vi "MasterAcquisitionFile_PCO_IOS_SingleWavelength.vi"() -> ()   [LabVIEW 2020]
uses:
  <userlib>/PCO LabVIEW 5.0.0/pco.camera/Controls/binning.ctl
  <vilib>/vision/driver/IMAQdx.llb/IMAQdx Camera Control Mode.ctl
  <vilib>/vision/driver/IMAQdx.llb/IMAQdx Acquisition Mode.ctl
  <vilib>/userDefined/High Color/IMAQdx.ctl
  <userlib>/PCO LabVIEW 5.0.0/pco.camera/Camera.lvclass
  <vilib>/vision/driver/IMAQdx.llb/IMAQdx Buffer Number Mode.ctl
  <vilib>/DAQmx/write.llb/DAQmx Write (Digital 1D Wfm NChan NSamp).vi
  <vilib>/DAQmx/read.llb/DAQmx Read (Analog 1D Wfm NChan NSamp).vi
  <vilib>/Waveform/DWDTOps.llb/DWDT Digital to Boolean Array.vi
  <vilib>/DAQmx/create/channels.llb/DAQmx Create Channel (CO-Pulse Generation-Frequency).vi
  <vilib>/DAQmx/configure/timing.llb/DAQmx Timing (Implicit).vi
  <vilib>/DAQmx/create/channels.llb/DAQmx Create Channel (AI-Voltage-Basic).vi
  <vilib>/DAQmx/configure/timing.llb/DAQmx Timing (Sample Clock).vi
  <vilib>/DAQmx/configure/trigger.llb/DAQmx Start Trigger (Digital Edge).vi
  <vilib>/DAQmx/create/channels.llb/DAQmx Create Channel (DO-Digital Output).vi
  <vilib>/Waveform/DWDTOps.llb/DWDT Boolean Array to Digital.vi
  <vilib>/Waveform/DWDTOps.llb/DWDT Uncompress Digital.vi
  <vilib>/DAQmx/miscellaneous.llb/DAQmx Fill In Error Info.vi
  <vilib>/vision/driver/NI_Vision_Acquisition_Software.lvlib
  <resource>/objmgr/imaqdx.rc
  <resource>/objmgr/daqmx.rc
panel:
  out "Recorded Images":u32
  in  "ROI":cluster{"x0":u64, "y0":u64, "x1":u64, "y1":u64}={"x0"=1, "y0"=1, "x1"=640, "y1"=540}
  in  "Binning":T1={"vert"=4, "horz"=4}
  in  "TriggerMode":T2(ring)=enum."external exposure start"
  in  "Exposure [s]":dbl=0.01 min=0.0005 max=2.0 step=0.001
  out "Image":T3(plugin-control)
  out "LED":bool
  out "Auditory":bool
  out "RPad":bool
  out "LPad":bool
  out "Finished":bool
  in  "Generate Stimuli":bool=TRUE
  in  "Sol Stim Parameters":cluster{"Fs":dbl, "Samples":dbl}
  in  "LED Stim Parameters":cluster{"Fs":dbl, "Samples":dbl}
  in  "Sol Duty Cycle (%)":dbl=50.0
  in  "Sol Freq":dbl=1.0
  in  "Sol Dur (s)":dbl=1.0
  in  "LED Duty Cycle (%)":dbl=10.0
  in  "LED Freq":dbl=10.0
  in  "LED Dur (s)":dbl=2.0
  out "Stimulus Order":digitalwaveform[](graph)=[{"t0"=timestamp(0 s since 1904-01-01), "dt"=5e-05, "Y"={"transitions"=[], "data"=array6001000x1[6001000 elements]}}, {"t0"=timestamp(0 s since 1904-01-01), "dt"=5e-05, "Y"={"transitions"=[], "data"=array6001000x1[6001000 elements]}}, {"t0"=timestamp(0 s since 1904-01-01), "dt"=5e-05, "Y"={"transitions"=[], "data"=array6001000x1[6001000 elements]}}, {"t0"=timestamp(0 s since 1904-01-01), "dt"=5e-05, "Y"={"transitions"=[], "data"=array6001000x1[6001000 elements]}}]
  out "Solenoid Stim":digitalwaveform(graph)={"t0"=timestamp(0 s since 1904-01-01), "dt"=5e-05, "Y"={"transitions"=[], "data"=array20000x1[20000 elements]}}
  in  "Trial Offset (s)":dbl=5.0
  in  "Interstim (s)":dbl=10.0
  in  "Right Pad":dbl=1.0
  in  "Left Pad":dbl=1.0
  in  "Auditory":dbl=1.0
  in  "LED":dbl
  out "?":T3(plugin-control)
  out "?":T3(plugin-control)
  out "?":T3(plugin-control)
  in  "stop":bool
  out "PCO":bool
  out "Pupil Cam":bool
  out "Whisk Cam":bool
  out "Web Cam":bool
  out "Analog":bool
  out "Web Cam Fs":dbl(knob) scale=0.0..200.0
  out "Whisk Cam Fs":dbl(knob) scale=0.0..200.0
  out "Last Whisk\nBuffer 2":u32=1
  out "Pupil Cam Fs":dbl(knob) scale=0.0..200.0
  out "Dropped 2":u32(slide) caption="Pupil Cam" scale=0.0..99.0
  out "Dev1 Samples":i32
  in  "Dev1 Analog Channels":string[](array[string])=["Cortical_LH", "Force_Sensor", "LPadSol", "RPadSol", "AudSol", "Hippocampus", "EMG", "Cortical_RH", "OptoLED"]
  in  "Analog Acquisition":cluster{"Analog Fs":u16}={"Analog Fs"=20000} {"Analog Fs" format="%0.0f"}
  in  "Sampling Rates":T4={"CBV Cam Fs"=30, "Whisk Cam Fs"=150, "Web Cam Fs"=30, "Pupil Cam Fs"=30}
  out "Notes Size":i32=8
  out "Notes Reversed":string[](array[string])=["Experimenter", "Animal ID", "Hemisphere", "Solenoid PSI", "Isoflurane time", "Session ID", "Amplifier Gain", "LED power (mW)"]
  out "Notes Array":string[](array[string])=["LED power (mW)", "Amplifier Gain", "Session ID", "Isoflurane time", "Solenoid PSI", "Hemisphere", "Animal ID", "Experimenter"]
  in  "Notes:":T5={"Experimenter"="Kevin", "Animal ID"="FS28", "Hemisphere"="LH", "Solenoid PSI"="10", "Isoflurane time"="1420", "Session ID"="Imaging Session One", "Amplifier Gain"="10000", "Opto LED (mW)"="10", "Wavelengths"="530 nm", "Lens mag"="1.5X"}
  in  "Target Path":path=path "D:/FS28/5 minute 530 only" caption="Final Save Location"
  out "Dropped":u32(slide) caption="Whisk Cam" scale=0.0..999.0
  out "Filename":string="230405_14_53_47"
  out "CBV Camera":bool=TRUE
  out "Time Elapsed (Min)":cluster{dbl, dbl}(slide)={15.0, 5.0010000000000004e-05} scale=0.0..15.0 scale format="%.1g"
  in  "Time (min)":dbl(knob)=15.0 min=0.5 max=20.0 step=0.5 scale=0.0..20.0 scale format="%#_2g"
  in  "Temp Path":path=path "D:/LabVIEW Streamed Data" caption="Temporary Path for Streamed Data"
  out "Last Whisk\nBuffer":u32=1
  # "PCO Parameters"
  # "Stimuli"
  # "LPAD"
  # "RPAD"
  # "AUD"
  # "LED"
  # "Dropped Frames"
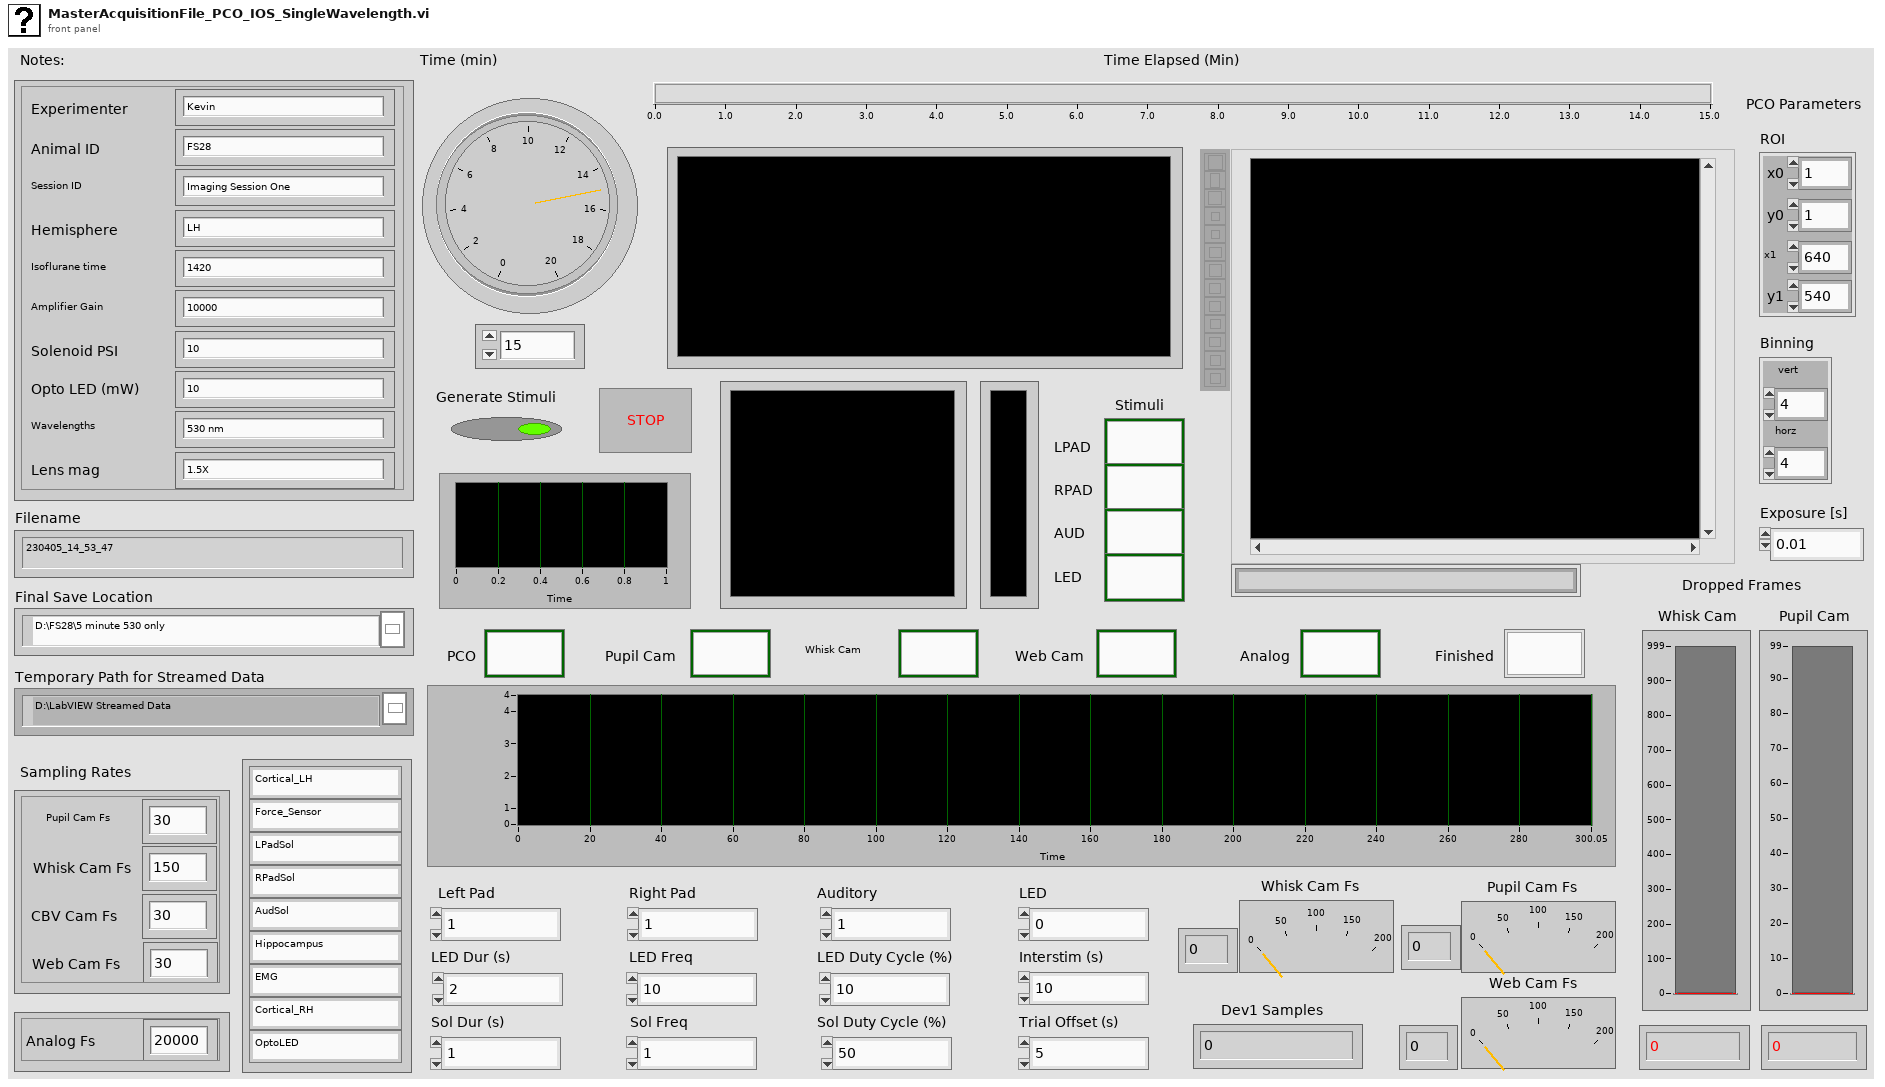
[diagram p1: front panel]
types:
  T1 = typedef "Camera.lvclass/binning.ctl" = cluster{"vert":u16, "horz":u16}
  T2 = enum16{"auto sequence", "software trigger", "external exposure start", "external exposure control"}
  T3 = typedef "IMAQ Image.ctl" = refnum<image>
  T4 = cluster{"CBV Cam Fs":u16, "Whisk Cam Fs":u16, "Web Cam Fs":u16, "Pupil Cam Fs":u16}
  T5 = cluster{"Experimenter":string, "Animal ID":string, "Hemisphere":string, "Solenoid PSI":string, "Isoflurane time":string, "Session ID":string, "Amplifier Gain":string, "Opto LED (mW)":string, "Wavelengths":string, "Lens mag":string}
  T6 = typedef "Image Type" = u32
  T7 = typedef "IMAQdx.ctl" = refnum<k21>
  T8 = enum16{"open", "replace", "create", "open or create", "replace or create", "replace or create with confirmation"}
  T9 = typedef "NI_Vision_Acquisition_Software.lvlib/IMAQdx Acquisition Mode.ctl" = enum32{"One Shot", "Continuous"}
  T10 = typedef "NI_Vision_Acquisition_Software.lvlib/IMAQdx Camera Control Mode.ctl" = enum32{"Controller", "Listener"}
  T11 = enum16{"open", "open or create", "create or replace", "create", "open (read-only)"}
  T12 = cluster{"exposure_time_s":dbl, "delay_time_s":dbl, "roi":cluster{"x0":u64, "y0":u64, "x1":u64, "y1":u64}, "timestamp_mode":u16, "pixelrate":u32, "trigger_mode":u16, "acquire_mode":u16, "metadata_mode":u16, "noisefilter_mode":u16, "binning":T1}
  T13 = typedef "IMAQ AVI2 Refnum.ctl" = refnum<k20>
  T14 = enum16{"sequence", "sequence non blocking", "ring buffer", "fifo", "sequence_dpcore", "sequence_non_blocking_dpcore", "ring_buffer_dpcore", "fifo_dpcore", "tif", "multitif", "pcoraw", "b16", "dicom", "multidicom"}
  T15 = enum16{"Undefined", "Mono8", "Mono16", "BGRA8", "RGBA8", "BGRA16", "RGBA16", "CompressedMono8"}
  T16 = enum16{"big-endian, network order", "native, host order", "little-endian"}
  T17 = typedef "NI_Vision_Acquisition_Software.lvlib/IMAQdx Buffer Number Mode.ctl" = enum32{"Next", "Last", "Buffer Number", "Every", "Last New"}
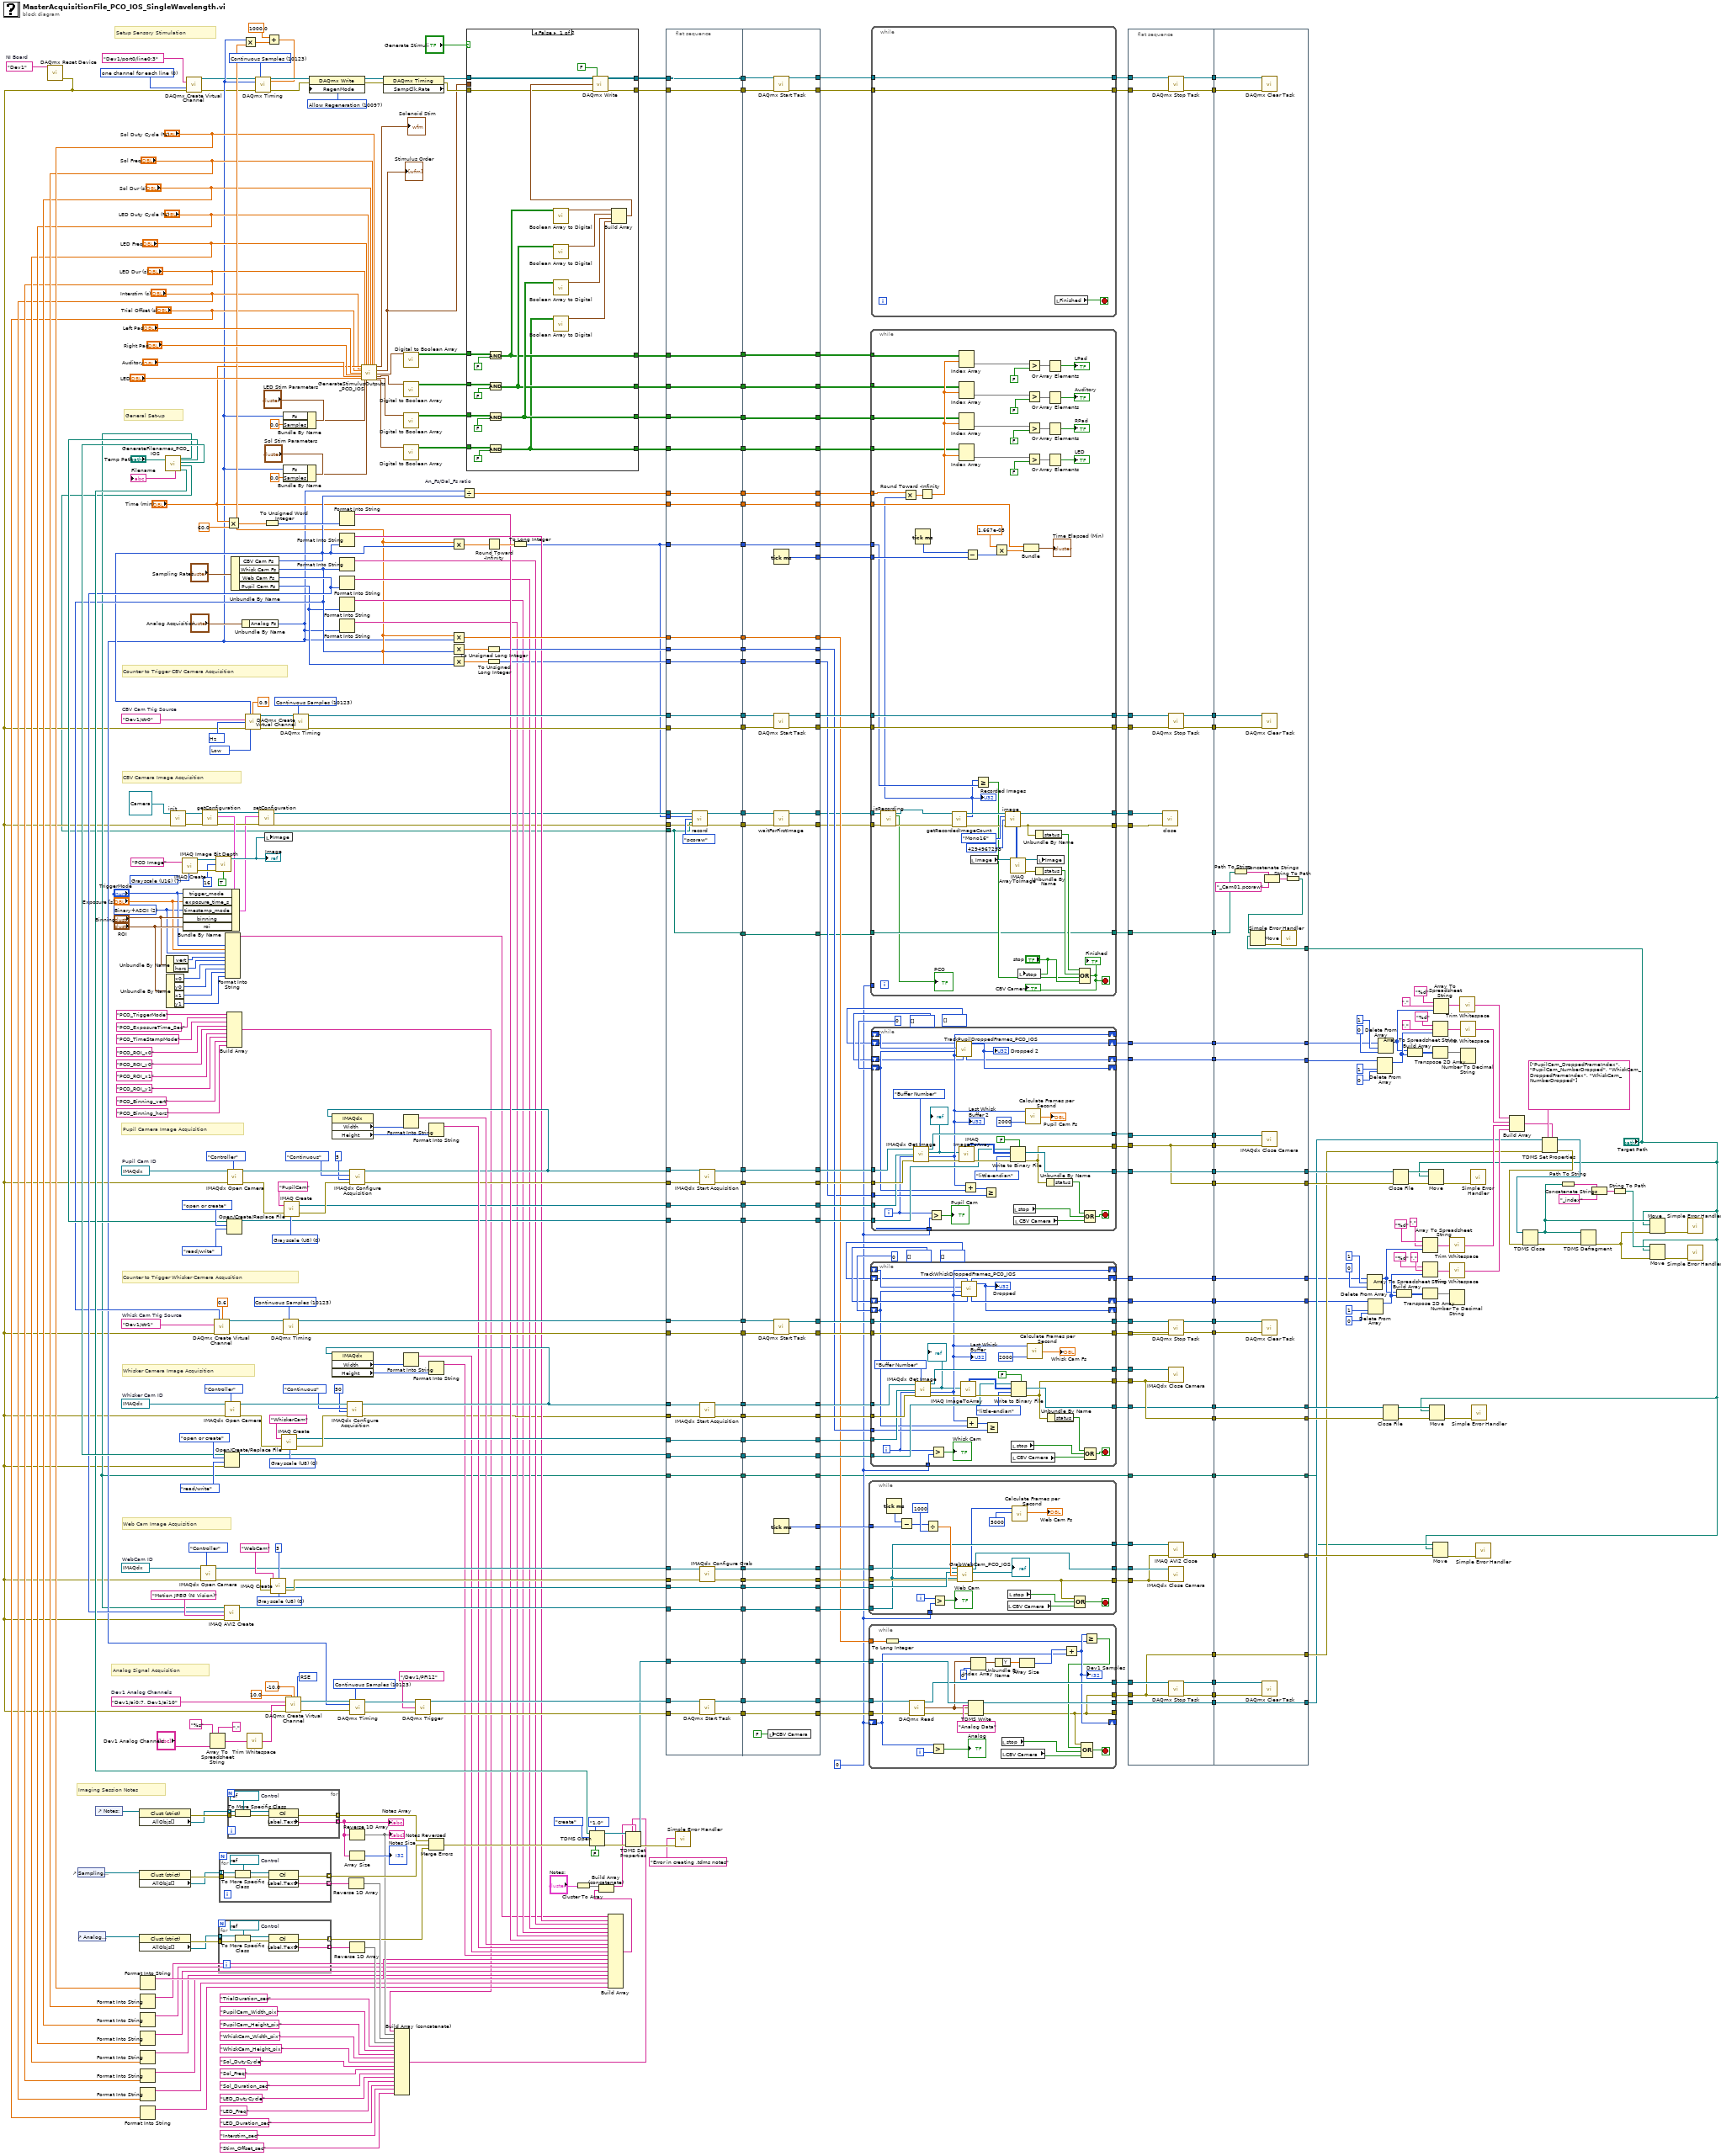
[diagram p0: block diagram]
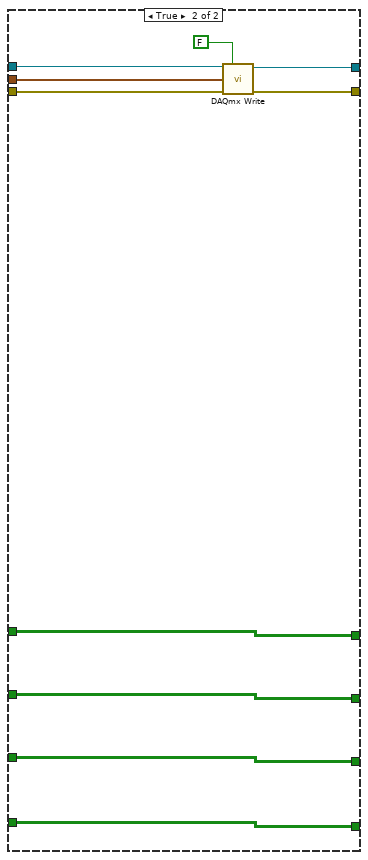
[diagram p2: hidden frame]
diagram:
  w24 = u16 2 items=["OFF", "Binary", "Binary+ASCII", "ASCII"] ("wTimeStampMode")
  w49 = T6 7 items=["Grayscale (U8)", "Grayscale (I16)", "Grayscale (SGL)", "Complex (CSG)", "RGB (U32)", "HSL (U32)", "RGB (U64)", "Grayscale (U16)"] ("Image Type")
  w141 = 10097 items=["Allow Regeneration"=10097, "Do Not Allow Regeneration"=10158] ("RegenMode")
  w142 = 10123 items=["Finite Samples"=10178, "Continuous Samples"=10123, "Hardware Timed Single Point"=12522] ("sample mode")
  w145 = 0 items=["one channel for each line", "one channel for all lines"] ("line grouping")
  w314 = tag "Dev1/ai0:7, Dev1/ai10"  # Dev1 Analog Channels
  w317 = T7 "cam3"  # WebCam ID
  w303 = T7 "cam1"  # Whisker Cam ID
  w441 = tag "Dev1/ctr1"  # Whisk Cam Trig Source
  w265 = T7 "cam2"  # Pupil Cam ID
  w107 = tag "Dev1/ctr0"  # CBV Cam Trig Source
  w268 = T6 0 items=["Grayscale (U8)", "Grayscale (I16)", "Grayscale (SGL)", "Complex (CSG)", "RGB (U32)", "HSL (U32)", "RGB (U64)", "Grayscale (U16)"] ("Image Type")
  w198 = 0
  w386 = 10123 items=["Finite Samples"=10178, "Continuous Samples"=10123, "Hardware Timed Single Point"=12522] ("sample mode")
  w389 = 10083 items=["default"=-1, "RSE"=10083, "NRSE"=10078, "Differential"=10106, "Pseudodifferential"=12529] ("input terminal configuration")
  w424 = T6 0 items=["Grayscale (U8)", "Grayscale (I16)", "Grayscale (SGL)", "Complex (CSG)", "RGB (U32)", "HSL (U32)", "RGB (U64)", "Grayscale (U16)"] ("Image Type")
  w431 = tag "Dev1"  # NI Board
  w432 = 10123 items=["Finite Samples"=10178, "Continuous Samples"=10123, "Hardware Timed Single Point"=12522] ("sample mode")
  w435 = 10373 items=["Hz"=10373] ("units")
  w436 = 10214 items=["High"=10192, "Low"=10214] ("idle state")
  w437 = 10123 items=["Finite Samples"=10178, "Continuous Samples"=10123, "Hardware Timed Single Point"=12522] ("sample mode")
  w444 = T6 0 items=["Grayscale (U8)", "Grayscale (I16)", "Grayscale (SGL)", "Complex (CSG)", "RGB (U32)", "HSL (U32)", "RGB (U64)", "Grayscale (U16)"] ("Image Type")
  # "General Set-up"
  # "Pupil Camera Image Acquisition"
  # "Whisker Camera Image Acquisition"
  # "Imaging Session Notes"
  # "Setup Sensory Stimulation"
  # "CBV Camera Image Acquisition"
  # "Counter to Trigger CBV Camera Acquisition"
  # "Counter to Trigger Whisker Camera Acqusition"
  # "Web Cam Image Acquisition"
  # "Analog Signal Acquisition"
  n1 = call <vilib>:"DAQmx Reset Device.vi"("device in"=w431) -> ("error out"=w39:errorcluster)  [unwired: 14 in]
  n2 = control-ref of="Sampling Rates"() -> (w323:refnum<vi>)
  n3 = control-ref of="Analog Acquisition"() -> (w322:refnum<vi>)
  n4 = control-ref of="Notes:"() -> (w344:refnum<vi>)
  n5 = property class="Clust (strict)"(reference=w344) -> (error out=w347:errorcluster, "AllObjs[]"=w281:refnum<vi>[])  [unwired: 1 in, 1 out]
  n6 = property class="Clust (strict)"(reference=w323) -> (error out=w342:errorcluster, "AllObjs[]"=w282:refnum<vi>[])  [unwired: 1 in, 1 out]
  n7 = property class="Clust (strict)"(reference=w322) -> (error out=w321:errorcluster, "AllObjs[]"=w280:refnum<vi>[])  [unwired: 1 in, 1 out]
  n8 = Format Into String("Sol Duty Cycle (%)") -> (resulting string=w175:string)  [unwired: 3 in, 1 out]
  n9 = Format Into String("Sol Freq") -> (resulting string=w174:string)  [unwired: 3 in, 1 out]
  n10 = Format Into String("Sol Dur (s)") -> (resulting string=w173:string)  [unwired: 3 in, 1 out]
  n11 = Format Into String("LED Duty Cycle (%)") -> (resulting string=w172:string)  [unwired: 3 in, 1 out]
  n12 = Format Into String("LED Freq") -> (resulting string=w171:string)  [unwired: 3 in, 1 out]
  n13 = Format Into String("LED Dur (s)") -> (resulting string=w170:string)  [unwired: 3 in, 1 out]
  n14 = Format Into String("Interstim (s)") -> (resulting string=w169:string)  [unwired: 3 in, 1 out]
  n15 = Format Into String("Trial Offset (s)") -> (resulting string=w168:string)  [unwired: 3 in, 1 out]
  n16 = call "GenerateFilenames_PCO_IOS.vi"("path"="Temp Path") -> ("TDMS Path"=w339:path, "PCO Path"=w5:path, "Basler Path"=w427:path, "WebCam Path"=w53:path, "Analog file name"=→"Filename":string, "Basler2 Path"=w264:path)  [unwired: 3 in, 2 out]
  n17 = Unbundle By Name("Binning") -> ("vert"=w23:u16, "horz"=w22:u16)
  n18 = Unbundle By Name("ROI") -> ("x0"=w21:u64, "y0"=w20:u64, "x1"=w19:u64, "y1"=w18:u64)
  n19 = call-dynamic "init.vi"("Camera in"=refnum<class "Camera.lvclass"> refnum ("PCOCamera in"), "error in (no error)"=w39) -> ("Camera out"=w42:refnum<class "Camera.lvclass">, "error out"=w41:errorcluster)  [unwired: 7 in]
  n20 = call "IMAQ Create"("Image Name"="PCO Image", "Image Type"=w49) -> ("New Image"=w48:T3, "error out"=w47:errorcluster)  [unwired: 3 in]
  n21 = call-poly <vilib>:"DAQmx Create Virtual Channel.vi"("lines"=tag "Dev1/port0/line0:3", "line grouping"=w145, "error in"=w39) -> ("task out"=w144:refnum<k21>, "error out"=w143:errorcluster)  [unwired: 11 in]
  n22 = call <vilib>:"IMAQdx Open Camera.vi"("Camera Control Mode"=IMAQdx_Camera_Control_Mode."Controller", "error in"=w39, "Session In"=w317) -> ("error out"=w420:errorcluster, "Session Out"=w418:T7)  [unwired: 7 in]
  n23 = call-dynamic "getConfiguration.vi"("error in (no error)"=w41, "Camera in"=w42) -> ("error out"=w40:errorcluster, "configuration"=w44:T12, "Camera out"=w43:refnum<class "Camera.lvclass">)  [unwired: 7 in]
  n24 = Bundle By Name(cluster=w44, "trigger_mode"="TriggerMode", "exposure_time_s"="Exposure [s]", "timestamp_mode"=w24, "binning"="Binning", "roi"="ROI") -> (w38:T12)
  n25 = Array To Spreadsheet String(delimiter (Tab)=",", array="Dev1 Analog Channels", 3:"%s" ("format string")) -> (spreadsheet string=w311:string)
  n26 = call "IMAQ Image Bit Depth"("Image"=w48, "Bit Depth (0)"=u32 16, "error in (no error)"=w47, "Get/Set Bit Depth? (Set)"=TRUE) -> ("Image Out"=w50:T3)  [unwired: 9 in, 2 out]
  "Image" <- w50
  n27 = for {
    tunnel: [w456] -> w319 mode=indexing
    tunnel: w321 -> [w455]
    tunnel: [w453] -> w320 mode=indexing
    tunnel: w280 -> [w452] mode=indexing
    w457 = refnum<vi> refnum  # Control
    n28 = To More Specific Class(target class=w457, reference=w452, error in=w455) -> (specific class reference=w458:refnum<vi>, error out=w454:errorcluster)
    n29 = property class="Ctl"(reference=w458, error in=w454) -> (error out=w453:errorcluster, "Label.Text"=w456:string)  [unwired: 1 out]
  }
  n30 = for {
    tunnel: [w463] -> w343 mode=indexing
    tunnel: w342 -> [w462]
    tunnel: [w460] -> w329 mode=indexing
    tunnel: w282 -> [w459] mode=indexing
    w464 = refnum<vi> refnum  # Control
    n31 = To More Specific Class(target class=w464, reference=w459, error in=w462) -> (specific class reference=w465:refnum<vi>, error out=w461:errorcluster)
    n32 = property class="Ctl"(reference=w465, error in=w461) -> (error out=w460:errorcluster, "Label.Text"=w463:string)  [unwired: 1 out]
  }
  n33 = Open/Create/Replace File(file path (use dialog)=w427, error in=w39, operation (0:open)=T8."open or create", access (0:read/write)=enum16{"read/write", "read-only", "write-only"}."read/write") -> (refnum out=w397:refnum<file>)  [unwired: 2 in, 2 out]
  n34 = Format Into String("TriggerMode", "Exposure [s]", w24, w23, w22, w21, w20, w19, w18) -> (resulting string=w16:string)  [unwired: 3 in, 1 out]
  n35 = call <vilib>:"IMAQdx Open Camera.vi"("Camera Control Mode"=IMAQdx_Camera_Control_Mode."Controller", "error in"=w39, "Session In"=w303) -> ("error out"=w447:errorcluster, "Session Out"=w450:T7)  [unwired: 7 in]
  n36 = Multiply(x="Time (min)", y=60.0) -> (x*y=w185:dbl)
  n37 = Build Array("PCO_TriggerMode", "PCO_ExposureTime_Sec", "PCO_TimeStampMode", "PCO_ROI_x0", "PCO_ROI_y0", "PCO_ROI_x1", "PCO_ROI_y1", "PCO_Binning_vert", "PCO_Binning_horz") -> (w17:string[])
  n38 = Open/Create/Replace File(file path (use dialog)=w264, operation (0:open)=T8."open or create", access (0:read/write)=enum16{"read/write", "read-only", "write-only"}."read/write") -> (refnum out=w249:refnum<file>)  [unwired: 3 in, 2 out]
  n39 = call <vilib>:"IMAQdx Open Camera.vi"("Camera Control Mode"=IMAQdx_Camera_Control_Mode."Controller", "error in"=w39, "Session In"=w265) -> ("error out"=w271:errorcluster, "Session Out"=w274:T7)  [unwired: 7 in]
  n40 = for {
    tunnel: [w470] -> w346 mode=indexing
    tunnel: w347 -> [w469]
    tunnel: [w467] -> w330 mode=indexing
    tunnel: w281 -> [w466] mode=indexing
    w471 = refnum<vi> refnum  # Control
    n41 = To More Specific Class(target class=w471, reference=w466, error in=w469) -> (specific class reference=w472:refnum<vi>, error out=w468:errorcluster)
    n42 = property class="Ctl"(reference=w472, error in=w468) -> (error out=w467:errorcluster, "Label.Text"=w470:string)  [unwired: 1 out]
  }
  "Notes Array" <- w346
  n43 = Unbundle By Name("Sampling Rates") -> ("CBV Cam Fs"=w186:u16, "Whisk Cam Fs"=w238:u16, "Web Cam Fs"=w316:u16, "Pupil Cam Fs"=w232:u16)
  n44 = call-poly <vilib>:"DAQmx Create Virtual Channel.vi"("frequency"=w238, "duty cycle"=0.6, "counter"=w441, "error in"=w39) -> ("task out"=w439:refnum<k21>, "error out"=w438:errorcluster)  [unwired: 10 in]
  n45 = call "IMAQ AVI2 Create"("error in (no error)"=w39, "Codec"="Motion JPEG (NI Vision)", "Frames Per Second"=w316, "AVI Path"=w53) -> ("AVI Refnum"=w410:T13)  [unwired: 6 in, 1 out]
  n46 = Unbundle By Name("Analog Acquisition") -> ("Analog Fs"=w158:u16)
  n47 = Multiply(x=w158, y=w185) -> (x*y=w118:dbl)
  n48 = call-poly <vilib>:"DAQmx Create Virtual Channel.vi"("frequency"=w186, "duty cycle"=0.9, "counter"=w107, "units"=w435, "error in"=w39, "idle state"=w436) -> ("task out"=w434:refnum<k21>, "error out"=w433:errorcluster)  [unwired: 8 in]
  n49 = call <vilib>:"Trim Whitespace.vi"("string"=w311) -> ("trimmed string"=w310:string)  [unwired: 1 in]
  n50 = call-dynamic "setConfiguration.vi"("error in (no error)"=w40, "configuration"=w38, "Camera in"=w43) -> ("error out"=w11:errorcluster, "Camera out"=w10:refnum<class "Camera.lvclass">)  [unwired: 7 in]
  n51 = To Unsigned Word Integer(number=w185) -> (unsigned 16bit integer=w306:u16)
  n52 = local write "Image"(w50) -> ()
  n53 = Add(x=1000.0, y=w118) -> (x+y=w116:dbl)
  n54 = call-poly <vilib>:"DAQmx Timing.vi"("task/channels in"=w144, "sample mode"=w142, "samples per channel"=w116, "rate"=w158, "error in"=w143) -> ("task out"=w138:refnum<k21>, "error out"=w137:errorcluster)  [unwired: 9 in]
  n55 = call "IMAQ Create"("Border Size"=3, "Image Name"="WebCam", "Image Type"=w424, "error in (no error)"=w420) -> ("New Image"=w417:T3, "error out"=w419:errorcluster)  [unwired: 1 in]
  n56 = call "IMAQ Create"("Image Name"="WhiskerCam", "Image Type"=w444, "error in (no error)"=w447) -> ("New Image"=w301:T3, "error out"=w445:errorcluster)  [unwired: 2 in]
  n57 = Bundle By Name(cluster="LED Stim Parameters", "Fs"=w158, "Samples"=0.0) -> (w191:cluster{"Fs":dbl, "Samples":dbl})
  n58 = Bundle By Name(cluster="Sol Stim Parameters", "Fs"=w158, "Samples"=0.0) -> (w192:cluster{"Fs":dbl, "Samples":dbl})
  n59 = call-poly <vilib>:"DAQmx Timing.vi"("task/channels in"=w439, "sample mode"=w437, "error in"=w438) -> ("task out"=w372:refnum<k21>, "error out"=w370:errorcluster)  [unwired: 11 in]
  n60 = call "IMAQ Create"("Image Name"="PupilCam", "Image Type"=w268, "error in (no error)"=w271) -> ("New Image"=w241:T3, "error out"=w269:errorcluster)  [unwired: 2 in]
  n61 = call-poly <vilib>:"DAQmx Create Virtual Channel.vi"("maximum value"=10.0, "minimum value"=-10.0, "input terminal configuration"=w389, "physical channels"=w314, "name to assign"=w310, "error in"=w39) -> ("task out"=w388:refnum<k21>, "error out"=w387:errorcluster)  [unwired: 8 in]
  n62 = call-poly <vilib>:"DAQmx Timing.vi"("task/channels in"=w434, "sample mode"=w432, "error in"=w433) -> ("task out"=w376:refnum<k21>, "error out"=w374:errorcluster)  [unwired: 11 in]
  n63 = property class="DAQmx Write"(reference=w138, error in=w137, "RegenMode"=w141) -> (reference out=w139:refnum<k21>, error out=w140:errorcluster)
  n64 = Format Into String(w306) -> (resulting string=w308:string)  [unwired: 3 in, 1 out]
  n65 = Format Into String(w186) -> (resulting string=w236:string)  [unwired: 3 in, 1 out]
  n66 = Format Into String(w238) -> (resulting string=w235:string)  [unwired: 3 in, 1 out]
  n67 = Format Into String(w316) -> (resulting string=w234:string)  [unwired: 3 in, 1 out]
  n68 = Format Into String(w232) -> (resulting string=w203:string)  [unwired: 3 in, 1 out]
  n69 = Format Into String(w158) -> (resulting string=w202:string)  [unwired: 3 in, 1 out]
  n70 = call <vilib>:"IMAQdx Configure Acquisition.vi"("error in"=w445, "Number of Buffers"=u32 50, "Continuous?"=IMAQdx_Acquisition_Mode."Continuous", "Session In"=w450) -> ("error out"=w210:errorcluster, "Session Out"=w302:T7)  [unwired: 6 in]
  n71 = property class="IMAQdx"(reference=w302) -> ("Width"=w305:u32, "Height"=w304:u32)  [unwired: 1 in, 2 out]
  n72 = Reverse 1D Array(array=w343) -> (reversed array=w333:string[])
  n73 = Reverse 1D Array(array=w346) -> (reversed array=w279:string[])
  "Notes Reversed" <- w279
  n74 = Array Size(array=w346) -> (size(s)=→"Notes Size":i32)
  n75 = Reverse 1D Array(array=w319) -> (reversed array=w318:string[])
  n76 = call <vilib>:"IMAQdx Configure Acquisition.vi"("error in"=w269, "Number of Buffers"=u32 5, "Continuous?"=IMAQdx_Acquisition_Mode."Continuous", "Session In"=w274) -> ("error out"=w251:errorcluster, "Session Out"=w242:T7)  [unwired: 6 in]
  n77 = property class="IMAQdx"(reference=w242) -> ("Width"=w263:u32, "Height"=w262:u32)  [unwired: 1 in, 2 out]
  n78 = call-poly <vilib>:"DAQmx Timing.vi"("task/channels in"=w388, "sample mode"=w386, "rate"=w158, "error in"=w387) -> ("task out"=w278:refnum<k21>, "error out"=w385:errorcluster)  [unwired: 10 in]
  n79 = call "GenerateStimulusOutputs_PCO_IOS.vi"("Trial duration (min)"="Time (min)", "Rest duration(s)"="Interstim (s)", "trial offset (s)"="Trial Offset (s)", "Left Pad"="Left Pad", "Right Pad"="Right Pad", "Auditory"="Auditory", "LED"="LED", "LED Stim Duration (s)"="LED Dur (s)", "LED Stim Parameters"=w191, "LED Frequency"="LED Freq", "Sol Stim Parameters"=w192, "LED duty cycle (%)"="LED Duty Cycle (%)", "Sol Stim Duration (s)"="Sol Dur (s)", "Sol Frequency"="Sol Freq", "Sol Duty Cycle (%)"="Sol Duty Cycle (%)") -> ("Solenoid Stim Waveforms"=→"Solenoid Stim":digitalwaveform, "Stimulus Digital Outputs"=w119:digitalwaveform[], "Left Pad Out"=w149:digitalwaveform, "Auditory Out"=w148:digitalwaveform, "Right Pad Out"=w147:digitalwaveform, "LED Out"=w146:digitalwaveform)  [unwired: 7 in]
  "Stimulus Order" <- w119
  n80 = property class="DAQmx Timing" props=["SampClk.Rate"](reference=w139, error in=w140) -> (reference out=w135:refnum<k21>, error out=w134:errorcluster)  [unwired: 1 out]
  n81 = Build Array (concatenate)(w17, w279, w333, w318, "TrialDuration_sec", "PupilCam_Width_pix", "PupilCam_Height_pix", "WhiskCam_Width_pix", "WhiskCam_Height_pix", "Sol_DutyCycle", "Sol_Freq", "Sol_Duration_sec", "LED_DutyCycle", "LED_Freq", "LED_Duration_sec", "Interstim_sec", "Stim_Offset_sec") -> (w276:string[])
  n82 = Format Into String(w263) -> (resulting string=w254:string)  [unwired: 3 in, 1 out]
  n83 = Format Into String(w305) -> (resulting string=w256:string)  [unwired: 3 in, 1 out]
  n84 = call-poly <vilib>:"Digital to Boolean Array.vi"("digital waveform"=w149) -> ("boolean array"=w127:bool[][])  [unwired: 9 in, 1 out]
  n85 = call-poly <vilib>:"Digital to Boolean Array.vi"("digital waveform"=w148) -> ("boolean array"=w126:bool[][])  [unwired: 9 in, 1 out]
  n86 = call-poly <vilib>:"Digital to Boolean Array.vi"("digital waveform"=w147) -> ("boolean array"=w125:bool[][])  [unwired: 9 in, 1 out]
  n87 = call-poly <vilib>:"Digital to Boolean Array.vi"("digital waveform"=w146) -> ("boolean array"=w124:bool[][])  [unwired: 9 in, 1 out]
  n88 = call-poly <vilib>:"DAQmx Trigger.vi"("task/channels in"=w278, "source"=tag "/Dev1/PFI12", "error in"=w385) -> ("task out"=w384:refnum<k21>, "error out"=w383:errorcluster)  [unwired: 11 in]
  n89 = Format Into String(w262) -> (resulting string=w255:string)  [unwired: 3 in, 1 out]
  n90 = Format Into String(w304) -> (resulting string=w257:string)  [unwired: 3 in, 1 out]
  n91 = Merge Errors(w330, w329, w320) -> (w328:errorcluster)
  n92 = Multiply(x=w185, y=w186) -> (x*y=w429:dbl)
  n93 = Multiply(x=w185, y=w158) -> (x*y=w292:dbl)
  n94 = Multiply(x=w238, y=w185) -> (x*y=w277:dbl)
  n95 = Multiply(x=w232, y=w185) -> (x*y=w237:dbl)
  n96 = Divide "An_Fs/Dal_Fs ratio"(x=w158, y=w186) -> (x/y=w102:dbl)
  n97 = case shown="False" "Generate Stimuli" {
    tunnel: w135 -> [w483 w504]
    tunnel: w134 -> [w482 w503]
    tunnel: [w480 w502] -> w132
    tunnel: [w481 w501] -> w130
    tunnel: w127 -> [w491 w500]
    tunnel: w126 -> [w492 w499]
    tunnel: w125 -> [w493 w498]
    tunnel: w124 -> [w494 w497]
    tunnel: [w475 w500] -> w123
    tunnel: [w476 w499] -> w122
    tunnel: [w477 w498] -> w121
    tunnel: [w473 w497] -> w120
    tunnel: w119 -> [_ w496]
    frame False {
      n98 = Compound Arithmetic op=AND(w491, FALSE) -> (w475:bool[][])
      n99 = Compound Arithmetic op=AND(w492, FALSE) -> (w476:bool[][])
      n100 = Compound Arithmetic op=AND(w493, FALSE) -> (w477:bool[][])
      n101 = Compound Arithmetic op=AND(w494, FALSE) -> (w473:bool[][])
      n102 = call-poly <vilib>:"Boolean Array to Digital.vi"("boolean array"=w475) -> ("digital waveform"=w485:digitalwaveform)  [unwired: 9 in, 1 out]
      n103 = call-poly <vilib>:"Boolean Array to Digital.vi"("boolean array"=w476) -> ("digital waveform"=w479:digitalwaveform)  [unwired: 9 in, 1 out]
      n104 = call-poly <vilib>:"Boolean Array to Digital.vi"("boolean array"=w477) -> ("digital waveform"=w478:digitalwaveform)  [unwired: 9 in, 1 out]
      n105 = call-poly <vilib>:"Boolean Array to Digital.vi"("boolean array"=w473) -> ("digital waveform"=w474:digitalwaveform)  [unwired: 9 in, 1 out]
      n106 = Build Array(w485, w479, w478, w474) -> (w484:digitalwaveform[])
      n107 = call-poly <vilib>:"DAQmx Write.vi"("task/channels in"=w483, "auto start"=FALSE, "data"=w484, "error in"=w482) -> ("task out"=w480:refnum<k21>, "error out"=w481:errorcluster)  [unwired: 9 in, 1 out]
    }
    frame True {
      n108 = call-poly <vilib>:"DAQmx Write.vi"("task/channels in"=w504, "auto start"=FALSE, "data"=w496, "error in"=w503) -> ("task out"=w502:refnum<k21>, "error out"=w501:errorcluster)  [unwired: 9 in, 1 out]
    }
  }
  n109 = To Unsigned Long Integer(number=w277) -> (unsigned 32bit integer=w290:u32)
  n110 = To Unsigned Long Integer(number=w237) -> (unsigned 32bit integer=w233:u32)
  n111 = Round Toward -Infinity(1:w429) -> (0:w428:dbl)
  n112 = To Long Integer(number=w428) -> (32bit integer=w9:i32)
  n113 = Cluster To Array(cluster="Notes:") -> (array=w340:string[])
  n114 = TDMS Open(6:FALSE ("disable buffering? (T)"), 7:enum16{"1.0", "2.0"}."1.0" ("file format version (2.0)"), 8:w328, 10:T11."create" ("operation (0:open)"), 11:w339) -> (0:w334:errorcluster, 3:w335:refnum<k34>)  [unwired: 2 in]
  n115 = Build Array(w16, w236, w235, w234, w203, w202, w308, w254, w255, w256, w257, w175, w174, w173, w172, w171, w170, w169, w168) -> (w315:string[])
  n116 = Build Array (concatenate)(w340, w315) -> (w332:string[])
  n117 = TDMS Set Properties(5:w332, 7:w276, 8:w334, 11:w335) -> (0:w327:errorcluster, 3:w331:refnum<k34>)  [unwired: 2 in, 2 out]
  n118 = flat-sequence {
    tunnel: w419 -> [w551]
    tunnel: w418 -> [w550]
    tunnel: w417 -> [w549]
    tunnel: [w549] -> w416
    tunnel: [w548] -> w414
    tunnel: [w547] -> w412
    tunnel: w410 -> [w546]
    tunnel: [w546] -> w409
    tunnel: w302 -> [w545]
    tunnel: w210 -> [w544]
    tunnel: [w543] -> w404
    tunnel: [w542] -> w402
    tunnel: [w541] -> w400
    tunnel: w301 -> [w541]
    tunnel: [w540] -> w398
    tunnel: w397 -> [w540]
    tunnel: w9 -> [w539]
    tunnel: [w539] -> w393
    tunnel: "Time (min)" -> [w538]
    tunnel: [w538] -> w390
    tunnel: w384 -> [w537]
    tunnel: w383 -> [w536]
    tunnel: [w535] -> w382
    tunnel: [w534] -> w381
    tunnel: [w533] -> w377
    tunnel: w331 -> [w533]
    tunnel: w376 -> [w532]
    tunnel: [w532] -> w375
    tunnel: w374 -> [w531]
    tunnel: [w531] -> w373
    tunnel: w372 -> [w530]
    tunnel: [w530] -> w371
    tunnel: w370 -> [w529]
    tunnel: [w529] -> w369
    tunnel: w292 -> [w528]
    tunnel: [w528] -> w291
    tunnel: w290 -> [w527]
    tunnel: [w527] -> w289
    tunnel: [w522] -> w253
    tunnel: w242 -> [w523]
    tunnel: [w520] -> w252
    tunnel: w251 -> [w521]
    tunnel: [w526] -> w250
    tunnel: w249 -> [w526]
    tunnel: w241 -> [w525]
    tunnel: [w525] -> w240
    tunnel: w233 -> [w524]
    tunnel: [w524] -> w231
    tunnel: [w519] -> w157
    tunnel: w123 -> [w519]
    tunnel: [w518] -> w156
    tunnel: w122 -> [w518]
    tunnel: [w517] -> w155
    tunnel: w121 -> [w517]
    tunnel: [w516] -> w154
    tunnel: w120 -> [w516]
    tunnel: [w515] -> w133
    tunnel: w132 -> [w515]
    tunnel: [w514] -> w131
    tunnel: w130 -> [w514]
    tunnel: w102 -> [w513]
    tunnel: [w513] -> w101
    tunnel: w53 -> [w512]
    tunnel: [w512] -> w54
    tunnel: [w511] -> w15
    tunnel: [w510] -> w14
    tunnel: w11 -> [w508]
    tunnel: w10 -> [w507]
    tunnel: w9 -> [w506]
    tunnel: w5 -> [w505]
    tunnel: [w505] -> w2
    tunnel: [w597] -> w421
    tunnel: w416 -> [w596]
    tunnel: [w596] -> w415
    tunnel: w414 -> [w595]
    tunnel: [w595] -> w413
    tunnel: w412 -> [w594]
    tunnel: [w594] -> w411
    tunnel: w409 -> [w593]
    tunnel: [w593] -> w408
    tunnel: [w578] -> w407
    tunnel: [w577] -> w406
    tunnel: [w592] -> w405
    tunnel: w404 -> [w592]
    tunnel: [w591] -> w403
    tunnel: w402 -> [w591]
    tunnel: [w590] -> w401
    tunnel: w400 -> [w590]
    tunnel: [w589] -> w399
    tunnel: w398 -> [w589]
    tunnel: [w582] -> w396
    tunnel: [w581] -> w395
    tunnel: [w588] -> w394
    tunnel: w393 -> [w587]
    tunnel: [w587] -> w392
    tunnel: [w586] -> w391
    tunnel: w390 -> [w586]
    tunnel: [w585] -> w379
    tunnel: w382 -> [w585]
    tunnel: [w584] -> w380
    tunnel: w381 -> [w584]
    tunnel: [w583] -> w200
    tunnel: w377 -> [w583]
    tunnel: w375 -> [w580]
    tunnel: w373 -> [w579]
    tunnel: w371 -> [w576]
    tunnel: w369 -> [w575]
    tunnel: w291 -> [w574]
    tunnel: [w574] -> w201
    tunnel: w289 -> [w573]
    tunnel: [w573] -> w230
    tunnel: w253 -> [w571]
    tunnel: w252 -> [w570]
    tunnel: w250 -> [w569]
    tunnel: [w571] -> w245
    tunnel: [w570] -> w244
    tunnel: [w569] -> w243
    tunnel: [w568] -> w239
    tunnel: w240 -> [w568]
    tunnel: [w567] -> w229
    tunnel: w231 -> [w567]
    tunnel: w157 -> [w563]
    tunnel: w156 -> [w566]
    tunnel: w155 -> [w565]
    tunnel: w154 -> [w564]
    tunnel: [w563] -> w153
    tunnel: [w566] -> w152
    tunnel: [w565] -> w151
    tunnel: [w564] -> w150
    tunnel: w133 -> [w562]
    tunnel: w131 -> [w561]
    tunnel: [w560] -> w129
    tunnel: [w559] -> w128
    tunnel: w101 -> [w558]
    tunnel: [w558] -> w100
    tunnel: [w557] -> w56
    tunnel: w54 -> [w557]
    tunnel: w15 -> [w556]
    tunnel: w14 -> [w555]
    tunnel: [w554] -> w13
    tunnel: [w553] -> w12
    tunnel: [w552] -> w1
    tunnel: w2 -> [w552]
    frame #0 {
      n119 = call-dynamic "record.vi"("Camera in"=w507, "num_images"=w506, "record_mode"=T14."pcoraw", "file_path"=w505, "error in (no error)"=w508) -> ("Camera out"=w511:refnum<class "Camera.lvclass">, "error out"=w510:errorcluster)  [unwired: 9 in]
      n120 = call <vilib>:"IMAQdx Start Acquisition.vi"("error in"=w521, "Session In"=w523) -> ("error out"=w520:errorcluster, "Session Out"=w522:T7)  [unwired: 8 in]
      n121 = call <vilib>:"IMAQdx Start Acquisition.vi"("error in"=w544, "Session In"=w545) -> ("error out"=w542:errorcluster, "Session Out"=w543:T7)  [unwired: 8 in]
      n122 = call <vilib>:"IMAQdx Configure Grab.vi"("error in"=w551, "Session In"=w550) -> ("error out"=w547:errorcluster, "Session Out"=w548:T7)  [unwired: 8 in]
      n123 = call <vilib>:"DAQmx Start Task.vi"("task/channels in"=w537, "error in"=w536) -> ("task out"=w535:refnum<k21>, "error out"=w534:errorcluster)  [unwired: 12 in]
    }
    frame #1 {
      n124 = local write "CBV Camera"(FALSE ("Finished Acquiring")) -> ()
      n125 = call-dynamic "waitForFirstImage.vi"("error in (no error)"=w555, "Camera in"=w556) -> ("error out"=w553:errorcluster, "Camera out"=w554:refnum<class "Camera.lvclass">)  [unwired: 8 in]
      n126 = call <vilib>:"DAQmx Start Task.vi"("task/channels in"=w562, "error in"=w561) -> ("task out"=w560:refnum<k21>, "error out"=w559:errorcluster)  [unwired: 12 in]
      n127 = Tick Count (ms)() -> (millisecond timer value=w588:u32)
      n128 = call <vilib>:"DAQmx Start Task.vi"("task/channels in"=w580, "error in"=w579) -> ("task out"=w582:refnum<k21>, "error out"=w581:errorcluster)  [unwired: 12 in]
      n129 = call <vilib>:"DAQmx Start Task.vi"("task/channels in"=w576, "error in"=w575) -> ("task out"=w578:refnum<k21>, "error out"=w577:errorcluster)  [unwired: 12 in]
      n130 = Tick Count (ms)() -> (millisecond timer value=w597:u32)
    }
  }
  n131 = call <vilib>:"Simple Error Handler.vi"("error source (\" \")"="Error in creating .tdms notes" ("error source (\" \")"), "error in (no error)"=w327) -> ()  [unwired: 3 in, 5 out]
  n132 = while {
    tunnel: w380 -> [w620]
    tunnel: w379 -> [w619]
    tunnel: w200 -> [w618]
    tunnel: [w617] -> w71
    tunnel: [w606] -> _
    tunnel: [w616] -> w99
    shift-right: [w610] -> _
    shift-left: w198 -> [w601]
    tunnel: [w606] -> w98
    tunnel: w201 -> [w604]
    i -> [w602]
    stop <- w607 stop-if-true
    n133 = To Long Integer(number=w604) -> (32bit integer=w605:i32)
    n134 = call-poly <vilib>:"DAQmx Read.vi"("task/channels in"=w619, "error in"=w620) -> ("task out"=w616:refnum<k21>, "data"=w598:waveform(dbl)[], "error out"=w609:errorcluster)  [unwired: 11 in]
    n135 = Greater?(x=w601, y=w602) -> (0:→"Analog":bool)
    n136 = TDMS Write(0:w618, 5:"Analog Data" ("group name in (Untitled)"), 9:w598, 11:w609) -> (4:w617:refnum<k34>, 15:w606:errorcluster)  [unwired: 2 in, 2 out]
    n137 = Index Array(array=w598, index=0) -> (element=w613:waveform(dbl))
    n138 = Unbundle By Name(w613) -> ("Y"=w612:dbl[])
    n139 = local read "CBV Camera"() -> (w600:bool)
    n140 = local read "stop"() -> (w599:bool)
    n141 = Array Size(array=w612) -> (size(s)=w611:i32)
    n142 = Add(x=w611, y=w601) -> (x+y=w610:i32)
    "Dev1 Samples" <- w610
    n143 = Greater Or Equal?(x=w610, y=w605) -> (x >= y?=w608:bool)
    n144 = Compound Arithmetic op=OR(w606, w608, w599, w600) -> (w607:bool)
  }
  n145 = while {
    tunnel: w421 -> [w637]
    tunnel: w415 -> [w635]
    tunnel: w413 -> [w634]
    tunnel: w411 -> [w633]
    tunnel: w408 -> [w631]
    tunnel: [w632] -> w90
    tunnel: [w623] -> w91
    tunnel: [w631] -> w89
    tunnel: w198 -> [w626]
    i -> [w627]
    stop <- w624 stop-if-true
    n146 = Tick Count (ms)() -> (millisecond timer value=w639:u32)
    n147 = Subtract(x=w639, y=w637) -> (x-y=w640:u32)
    n148 = Divide(x=w640, y=u32 1000) -> (x/y=w636:dbl)
    n149 = Greater?(x=w627, y=w626) -> (0:→"Web Cam":bool)
    n150 = call "GrabWebCam_PCO_IOS.vi"("Session In"=w634, "Image In"=w635, "Trial Time"=w636, "AVI Refnum"=w631, "error in"=w633) -> ("Session Out"=w632:T7, "WebCam Img Out"=→"?":T3, "Buffer Number Out"=w630:u32, "error out"=w623:errorcluster)  [unwired: 7 in]
    n151 = local read "CBV Camera"() -> (w625:bool)
    n152 = local read "stop"() -> (w622:bool)
    n153 = call <vilib>:"Calculate Frames per Second.vi"("Update Interval (ms)"=u32 5000, "Buffer Number"=w630) -> ("Processed Frames/s"=→"Web Cam Fs":dbl)  [unwired: 7 in, 2 out]
    n154 = Compound Arithmetic op=OR(w623, w622, w625) -> (w624:bool)
  }
  n155 = while {
    tunnel: [w693] -> w111
    tunnel: w396 -> [w693]
    tunnel: [w692] -> w110
    tunnel: w395 -> [w692]
    tunnel: w394 -> [w691]
    tunnel: w392 -> [w647]
    tunnel: w391 -> [w690]
    tunnel: w198 -> [_]
    tunnel: w153 -> [w674]
    tunnel: w152 -> [w675]
    tunnel: w151 -> [w669]
    tunnel: w150 -> [w666]
    tunnel: w100 -> [w663]
    tunnel: w13 -> [w662]
    tunnel: w12 -> [w661]
    tunnel: [w651] -> w8
    tunnel: [w650] -> w7
    tunnel: [w643] -> w4
    tunnel: w1 -> [w643]
    stop <- w685 stop-if-true
    n156 = call-dynamic "isRecording.vi"("Camera in"=w662, "error in (no error)"=w661) -> ("Camera out"=w649:refnum<class "Camera.lvclass">, "recording"=→"PCO":bool, "error out"=w648:errorcluster)  [unwired: 11 in]
    n157 = Tick Count (ms)() -> (millisecond timer value=w696:u32)
    n158 = call-dynamic "getRecordedImageCount.vi"("Camera in"=w649, "error in (no error)"=w648) -> ("Camera out"=w655:refnum<class "Camera.lvclass">, "recorded_image_count"=w646:u32, "error out"=w654:errorcluster)  [unwired: 11 in]
    "Recorded Images" <- w646
    n159 = Multiply(x=w663, y=w646) -> (x*y=w686:dbl)
    n160 = Round Toward -Infinity(1:w686) -> (0:w680:dbl)
    n161 = Index Array(array=w674, index (row)=w680) -> (element=w673:bool[])  [unwired: 1 in]
    n162 = Index Array(array=w675, index (row)=w680) -> (element=w671:bool[])  [unwired: 1 in]
    n163 = Index Array(array=w669, index (row)=w680) -> (element=w668:bool[])  [unwired: 1 in]
    n164 = Index Array(array=w666, index (row)=w680) -> (element=w665:bool[])  [unwired: 1 in]
    n165 = Subtract(x=w696, y=w691) -> (x-y=w695:u32)
    n166 = local read "Image"() -> (w660:T3)
    n167 = Greater Or Equal?(x=w646, y=w647) -> (x >= y?=w652:bool)
    n168 = Multiply(x=w695, y=1.667e-05) -> (x*y=w694:dbl)
    n169 = call-dynamic "image.vi"("Camera in"=w655, "data_format"=T15."Mono16", "image_index"=u32 4294967295 ("dwImgIdx"), "error in (no error)"=w654) -> ("Camera out"=w651:refnum<class "Camera.lvclass">, "raw_image (U16)"=w659:u16[][], "error out"=w650:errorcluster)  [unwired: 4 in, 5 out]
    n170 = call "IMAQ ArrayToImage"("Image Pixels (U16)"=w659, "Image"=w660) -> ("error out"=w657:errorcluster, "Image Out"=w653:T3)  [unwired: 8 in]
    n171 = local write "stop"("stop") -> ()
    n172 = Bundle("Time (min)"=w690, w694) -> (→"Time Elapsed (Min)":cluster{"Time (min)":dbl, dbl})  [unwired: 1 in]
    n173 = Greater?(x=w673, y=FALSE ("Boolean")) -> (0:w672:bool[])
    n174 = Greater?(x=w671, y=FALSE ("Boolean")) -> (0:w670:bool[])
    n175 = Greater?(x=w668, y=FALSE ("Boolean")) -> (0:w667:bool[])
    n176 = Greater?(x=w665, y=FALSE ("Boolean")) -> (0:w664:bool[])
    n177 = Unbundle By Name(w650) -> ("status"=w644:bool)
    n178 = Unbundle By Name(w657) -> ("status"=w645:bool)
    n179 = local write "Image"(w653) -> ()
    n180 = Or Array Elements(Boolean array=w672) -> (logical OR=→"LPad":bool)
    n181 = Or Array Elements(Boolean array=w670) -> (logical OR=→"Auditory":bool)
    n182 = Or Array Elements(Boolean array=w667) -> (logical OR=→"RPad":bool)
    n183 = Or Array Elements(Boolean array=w664) -> (logical OR=→"LED":bool)
    n184 = Compound Arithmetic op=OR(w644, w645, w652, "stop") -> (w685:bool)
    "CBV Camera" <- w685
    "Finished" <- w685
  }
  n185 = while {
    tunnel: w407 -> [w723]
    tunnel: [w724] -> w94
    tunnel: w406 -> [w724]
    tunnel: [w723] -> w95
    tunnel: [w716] -> w85
    tunnel: [w717] -> w86
    tunnel: [w722] -> w81
    tunnel: w405 -> [w721]
    tunnel: w403 -> [w720]
    tunnel: w401 -> [w719]
    tunnel: w399 -> [w718]
    shift-right: [w707] -> _
    shift-left: _ -> [w705]
    shift-right: [w702] -> _
    shift-left: u32 0 ("New Lost") -> [w706]
    shift-right: [w703] -> w66
    shift-left: u32[] [] ("NewBuffNum") -> [w704]
    shift-right: [w709] -> w69
    shift-left: u32[] [] ("NewNumLost") -> [w708]
    tunnel: w230 -> [w714]
    tunnel: w198 -> [w710]
    i -> [w697]
    stop <- w713 stop-if-true
    n186 = call <vilib>:"IMAQdx Get Image.vi"("Buffer Number Mode (Next)"=IMAQdx_Buffer_Number_Mode."Buffer Number", "error in"=w720, "Buffer Number In"=w697, "Image In"=w719, "Session In"=w721) -> ("error out"=w730:errorcluster, "Buffer Number Out"=w707:u32, "Image Out"=w699:T3, "Session Out"=w716:T7)  [unwired: 3 in]
    "Last Whisk\nBuffer" <- w707
    "?" <- w699
    n187 = Greater?(x=w697, y=w710) -> (0:→"Whisk Cam":bool)
    n188 = call "IMAQ ImageToArray"("error in (no error)"=w730, "Image"=w699) -> ("error out"=w729:errorcluster, "Image Pixels (U8)"=w728:u8[][])  [unwired: 2 in, 3 out]
    n189 = call "TrackWhiskDroppedFrames_PCO_IOS.vi"("NumLost"=w708, "BuffNum"=w704, "Curr Buffer"=w707, "Prev Lost"=w706, "Prev Buffer"=w705) -> ("New Lost"=w702:u32, "NewNumLost"=w709:u32[], "NewBuffNum"=w703:u32[])  [unwired: 4 in]
    "Dropped" <- w702
    n190 = Add(x=w707, y=w706) -> (x+y=w715:u32)
    n191 = Greater Or Equal?(x=w715, y=w714) -> ()  [unwired: 1 out]
    n192 = Write to Binary File(file (use dialog)=w718, data=w728, error in=w729, 5:FALSE ("prepend array or string size? (T)"), 9:T16."little-endian" ("byte order (0:big-endian, network order)")) -> (refnum out=w722:refnum<file>, error out=w717:errorcluster)  [unwired: 1 in, 1 out]
    n193 = local read "stop"() -> (w701:bool)
    n194 = local read "CBV Camera"() -> (w700:bool)
    n195 = call <vilib>:"Calculate Frames per Second.vi"("Update Interval (ms)"=u32 2000, "Buffer Number"=w707) -> ("Processed Frames/s"=→"Whisk Cam Fs":dbl)  [unwired: 7 in, 2 out]
    n196 = Unbundle By Name(w717) -> ("status"=w698:bool)
    n197 = Compound Arithmetic op=OR(w698, w701, w700) -> (w713:bool)
  }
  n198 = while {
    tunnel: w129 -> [w732]
    tunnel: [w733] -> w114
    tunnel: w128 -> [w733]
    tunnel: [w732] -> w115
    stop <- w734 stop-if-true
    n199 = local read "Finished"() -> (w734:bool)
  }
  n200 = while {
    tunnel: [w749] -> w105
    tunnel: [w750] -> w104
    tunnel: [w759] -> w79
    tunnel: w245 -> [w758]
    tunnel: w244 -> [w757]
    tunnel: w239 -> [w756]
    tunnel: w243 -> [w755]
    shift-right: [w748] -> _
    shift-left: _ -> [w754]
    shift-right: [w753] -> _
    shift-left: u32 0 ("New Lost") -> [w747]
    shift-right: [w752] -> w60
    shift-left: u32[] [] ("NewBuffNum") -> [w743]
    shift-right: [w751] -> w63
    shift-left: u32[] [] ("NewNumLost") -> [w744]
    tunnel: w229 -> [w742]
    tunnel: w198 -> [w740]
    i -> [w735]
    stop <- w745 stop-if-true
    n201 = call <vilib>:"IMAQdx Get Image.vi"("Buffer Number Mode (Next)"=IMAQdx_Buffer_Number_Mode."Buffer Number", "error in"=w757, "Buffer Number In"=w735, "Image In"=w756, "Session In"=w758) -> ("error out"=w766:errorcluster, "Buffer Number Out"=w748:u32, "Image Out"=w737:T3, "Session Out"=w749:T7)  [unwired: 3 in]
    "Last Whisk\nBuffer 2" <- w748
    "?" <- w737
    n202 = Greater?(x=w735, y=w740) -> (0:→"Pupil Cam":bool)
    n203 = call "TrackPupilDroppedFrames_PCO_IOS.vi"("NumLost"=w744, "BuffNum"=w743, "Curr Buffer"=w748, "Prev Lost"=w747, "Prev Buffer"=w754) -> ("New Lost"=w753:u32, "NewNumLost"=w751:u32[], "NewBuffNum"=w752:u32[])  [unwired: 4 in]
    "Dropped 2" <- w753
    n204 = call "IMAQ ImageToArray"("error in (no error)"=w766, "Image"=w737) -> ("error out"=w765:errorcluster, "Image Pixels (U8)"=w764:u8[][])  [unwired: 2 in, 3 out]
    n205 = Add(x=w748, y=w747) -> (x+y=w746:u32)
    n206 = Greater Or Equal?(x=w746, y=w742) -> ()  [unwired: 1 out]
    n207 = Write to Binary File(file (use dialog)=w755, data=w764, error in=w765, 5:FALSE ("prepend array or string size? (T)"), 9:T16."little-endian" ("byte order (0:big-endian, network order)")) -> (refnum out=w759:refnum<file>, error out=w750:errorcluster)  [unwired: 1 in, 1 out]
    n208 = local read "stop"() -> (w739:bool)
    n209 = local read "CBV Camera"() -> (w738:bool)
    n210 = call <vilib>:"Calculate Frames per Second.vi"("Update Interval (ms)"=u32 2000, "Buffer Number"=w748) -> ("Processed Frames/s"=→"Pupil Cam Fs":dbl)  [unwired: 7 in, 2 out]
    n211 = Unbundle By Name(w750) -> ("status"=w736:bool)
    n212 = Compound Arithmetic op=OR(w736, w739, w738) -> (w745:bool)
  }
  n213 = flat-sequence {
    tunnel: w115 -> [w802]
    tunnel: w114 -> [w801]
    tunnel: [w800] -> w113
    tunnel: [w799] -> w112
    tunnel: w111 -> [w798]
    tunnel: w110 -> [w797]
    tunnel: [w796] -> w109
    tunnel: [w795] -> w108
    tunnel: [w794] -> w106
    tunnel: w105 -> [w794]
    tunnel: w104 -> [w778]
    tunnel: [w778] -> w103
    tunnel: w99 -> [w793]
    tunnel: w98 -> [w777]
    tunnel: [w792] -> w97
    tunnel: [w791] -> w96
    tunnel: w95 -> [w790]
    tunnel: w94 -> [w789]
    tunnel: [w788] -> _
    tunnel: [w787] -> _
    tunnel: [w788] -> w93
    tunnel: [w787] -> w92
    tunnel: w91 -> [w785]
    tunnel: w90 -> [w786]
    tunnel: w89 -> [w784]
    tunnel: [w783] -> w88
    tunnel: w86 -> [w781]
    tunnel: w85 -> [w782]
    tunnel: [w781] -> w83
    tunnel: [w780] -> w82
    tunnel: w81 -> [w780]
    tunnel: w79 -> [w779]
    tunnel: [w779] -> w78
    tunnel: [w778] -> w75
    tunnel: [w777] -> w74
    tunnel: w71 -> [w776]
    tunnel: [w776] -> w72
    tunnel: w69 -> [w775]
    tunnel: [w775] -> w68
    tunnel: w66 -> [w774]
    tunnel: [w774] -> w65
    tunnel: w63 -> [w773]
    tunnel: [w773] -> w62
    tunnel: w60 -> [w772]
    tunnel: [w772] -> w59
    tunnel: w56 -> [w771]
    tunnel: [w771] -> w55
    tunnel: w8 -> [w770]
    tunnel: w7 -> [w769]
    tunnel: w4 -> [w768]
    tunnel: [w768] -> w3
    tunnel: w113 -> [w831]
    tunnel: w112 -> [w830]
    tunnel: w109 -> [w829]
    tunnel: w108 -> [w828]
    tunnel: w106 -> [w827]
    tunnel: w103 -> [w826]
    tunnel: w97 -> [w825]
    tunnel: w96 -> [w824]
    tunnel: w93 -> [w823]
    tunnel: w92 -> [w822]
    tunnel: w88 -> [w821]
    tunnel: [w821] -> w87
    tunnel: [w820] -> w84
    tunnel: w83 -> [w820]
    tunnel: w82 -> [w819]
    tunnel: [w819] -> w80
    tunnel: w78 -> [w818]
    tunnel: [w818] -> w77
    tunnel: [w817] -> w76
    tunnel: w75 -> [w817]
    tunnel: w74 -> [w816]
    tunnel: [w816] -> w73
    tunnel: w72 -> [w815]
    tunnel: [w815] -> w70
    tunnel: w68 -> [w814]
    tunnel: [w814] -> w67
    tunnel: [w813] -> w64
    tunnel: w65 -> [w813]
    tunnel: w62 -> [w812]
    tunnel: [w812] -> w61
    tunnel: w59 -> [w811]
    tunnel: [w811] -> w58
    tunnel: [w810] -> w57
    tunnel: w55 -> [w810]
    tunnel: "Target Path" -> [w808]
    tunnel: w3 -> [w804]
    frame #0 {
      n214 = call-dynamic "close.vi"("error in (no error)"=w769, "Camera in"=w770) -> ()  [unwired: 9 in, 1 out]
      n215 = call <vilib>:"DAQmx Stop Task.vi"("task/channels in"=w802, "error in"=w801) -> ("task out"=w800:refnum<k21>, "error out"=w799:errorcluster)  [unwired: 12 in]
      n216 = call <vilib>:"DAQmx Stop Task.vi"("task/channels in"=w798, "error in"=w797) -> ("task out"=w796:refnum<k21>, "error out"=w795:errorcluster)  [unwired: 12 in]
      n217 = call <vilib>:"DAQmx Stop Task.vi"("task/channels in"=w790, "error in"=w789) -> ("task out"=w788:refnum<k21>, "error out"=w787:errorcluster)  [unwired: 12 in]
      n218 = call <vilib>:"IMAQdx Close Camera.vi"("error in"=w781, "Session In"=w782) -> ()  [unwired: 9 in, 1 out]
      n219 = call "IMAQ AVI2 Close"("error in (no error)"=w785, "AVI Refnum"=w784) -> ("error out"=w783:errorcluster)  [unwired: 9 in]
      n220 = call <vilib>:"IMAQdx Close Camera.vi"("error in"=w785, "Session In"=w786) -> ()  [unwired: 9 in, 1 out]
      n221 = call <vilib>:"DAQmx Stop Task.vi"("task/channels in"=w793, "error in"=w777) -> ("task out"=w792:refnum<k21>, "error out"=w791:errorcluster)  [unwired: 12 in]
    }
    frame #1 {
      n222 = Path To String(path=w804) -> (string=w807:string)
      n223 = call <vilib>:"DAQmx Clear Task.vi"("task in"=w831, "error in"=w830) -> ()  [unwired: 13 in, 1 out]
      n224 = call <vilib>:"DAQmx Clear Task.vi"("task in"=w829, "error in"=w828) -> ()  [unwired: 13 in, 1 out]
      n225 = call <vilib>:"IMAQdx Close Camera.vi"("error in"=w826, "Session In"=w827) -> ()  [unwired: 9 in, 1 out]
      n226 = call <vilib>:"DAQmx Clear Task.vi"("task in"=w823, "error in"=w822) -> ()  [unwired: 13 in, 1 out]
      n227 = call <vilib>:"DAQmx Clear Task.vi"("task in"=w825, "error in"=w824) -> ()  [unwired: 13 in, 1 out]
      n228 = Concatenate Strings(w807, "_Cam01.pcoraw" ("string")) -> (w805:string)
      n229 = String To Path(string=w805) -> (path=w803:path)
      n230 = Move(source path=w803, 10:w808) -> (error out=w809:errorcluster)  [unwired: 3 in, 2 out]
      n231 = call <vilib>:"Simple Error Handler.vi"("error in (no error)"=w809) -> ()  [unwired: 1 in, 8 out]
    }
  }
  n232 = Delete From Array(array=w64, length=1, index=0) -> (array with subset deleted=w284:u32[])  [unwired: 1 out]
  n233 = Delete From Array(array=w67, length=1, index=0) -> (array with subset deleted=w285:u32[])  [unwired: 1 out]
  n234 = Delete From Array(array=w61, length=1, index=0) -> (array with subset deleted=w216:u32[])  [unwired: 1 out]
  n235 = Delete From Array(array=w58, length=1, index=0) -> (array with subset deleted=w215:u32[])  [unwired: 1 out]
  n236 = Close File(refnum=w80, error in=w84) -> (path=w360:path, error out=w359:errorcluster)
  n237 = Close File(refnum=w77, error in=w76) -> (path=w212:path, error out=w211:errorcluster)
  n238 = Build Array(w284, w285) -> (w287:u32[][])
  n239 = Build Array(w215, w216) -> (w218:u32[][])
  n240 = Array To Spreadsheet String(delimiter (Tab)=",", array=w285, 3:"%d" ("format string")) -> (spreadsheet string=w293:string)
  n241 = Transpose 2D Array(2D array=w287) -> (transposed array=w286:u32[][])
  n242 = Array To Spreadsheet String(delimiter (Tab)=",", array=w284, 3:"%d" ("format string")) -> (spreadsheet string=w294:string)
  n243 = Move(source path=w212, error in=w211, 10:"Target Path") -> (error out=w213:errorcluster)  [unwired: 2 in, 2 out]
  n244 = Move(source path=w360, error in=w359, 10:"Target Path") -> (error out=w357:errorcluster)  [unwired: 2 in, 2 out]
  n245 = Array To Spreadsheet String(delimiter (Tab)=",", array=w216, 3:"%d" ("format string")) -> (spreadsheet string=w219:string)
  n246 = Transpose 2D Array(2D array=w218) -> (transposed array=w217:u32[][])
  n247 = Move(source path=w57, error in=w87, 10:"Target Path") -> (error out=w356:errorcluster)  [unwired: 2 in, 2 out]
  n248 = Array To Spreadsheet String(delimiter (Tab)=",", array=w215, 3:"%d" ("format string")) -> (spreadsheet string=w220:string)
  n249 = call <vilib>:"Trim Whitespace.vi"("string"=w294) -> ("trimmed string"=w206:string)  [unwired: 1 in]
  n250 = call <vilib>:"Trim Whitespace.vi"("string"=w293) -> ("trimmed string"=w205:string)  [unwired: 1 in]
  n251 = Number To Decimal String(number=w286) -> ()  [unwired: 1 in, 1 out]
  n252 = call <vilib>:"Trim Whitespace.vi"("string"=w220) -> ("trimmed string"=w207:string)  [unwired: 1 in]
  n253 = call <vilib>:"Trim Whitespace.vi"("string"=w219) -> ("trimmed string"=w208:string)  [unwired: 1 in]
  n254 = Number To Decimal String(number=w217) -> ()  [unwired: 1 in, 1 out]
  n255 = call <vilib>:"Simple Error Handler.vi"("error in (no error)"=w213) -> ()  [unwired: 1 in, 8 out]
  n256 = call <vilib>:"Simple Error Handler.vi"("error in (no error)"=w357) -> ()  [unwired: 1 in, 8 out]
  n257 = call <vilib>:"Simple Error Handler.vi"("error in (no error)"=w356) -> ()  [unwired: 1 in, 8 out]
  n258 = Build Array(w207, w208, w206, w205) -> (w204:string[])
  n259 = TDMS Set Properties(5:w204, 7:string[] ["PupilCam_DroppedFrameIndex", "PupilCam_NumberDropped", "WhiskCam_DroppedFrameIndex", "WhiskCam_NumberDropped"] ("channel name(s) in (Untitled)"), 8:w73, 11:w70) -> (0:w300:errorcluster, 3:w299:refnum<k34>)  [unwired: 2 in, 2 out]
  n260 = TDMS Close(8:w300, 11:w299) -> (0:w361:errorcluster, 3:w353:path)
  n261 = Path To String(path=w353) -> (string=w355:string)
  n262 = TDMS Defragment(4:w361, 7:w353) -> (0:w350:errorcluster)
  n263 = Concatenate Strings(w355, "_index" ("string")) -> (w352:string)
  n264 = String To Path(string=w352) -> (path=w351:path)
  n265 = Move(source path=w353, error in=w350, 10:"Target Path") -> (error out=w358:errorcluster)  [unwired: 2 in, 2 out]
  n266 = Move(source path=w351, error in=w350, 10:"Target Path") -> (error out=w214:errorcluster)  [unwired: 2 in, 2 out]
  n267 = call <vilib>:"Simple Error Handler.vi"("error in (no error)"=w358) -> ()  [unwired: 1 in, 8 out]
  n268 = call <vilib>:"Simple Error Handler.vi"("error in (no error)"=w214) -> ()  [unwired: 1 in, 8 out]
